vi "Read Subscribe request data JSON.vi"(8 "error in (no error)":errorcluster, 11 "Subscribe JSON in":refnum<class "Subscribe JSON.lvclass">) -> (0 "error out":errorcluster, 2 "Subscribe request data (JSON)":T1={"Topic"="", "Subscribe result notifer"=refnum, "Options"="{}"}, 3 "Subscribe JSON out":refnum<class "Subscribe JSON.lvclass">)   [LabVIEW 2020, in "wamplv.lvlib" / "Subscribe JSON.lvclass"]
uses:
  Subscribe JSON.lvclass
  Subscribe JSON.lvclass/Subscribe JSON.ctl
  WAMP Client/Private/TypeDef/EVENT payload (JSON).ctl
  wamplv.lvlib
  WAMP Client/API/TypeDefs/Error or abort detail (JSON).ctl
  WAMP Client/API/TypeDefs/Combined error.ctl
  Subscribe result (JSON).ctl
  WAMP Client/Private/TypeDef/SUBSCRIBE Request Data (JSON).ctl
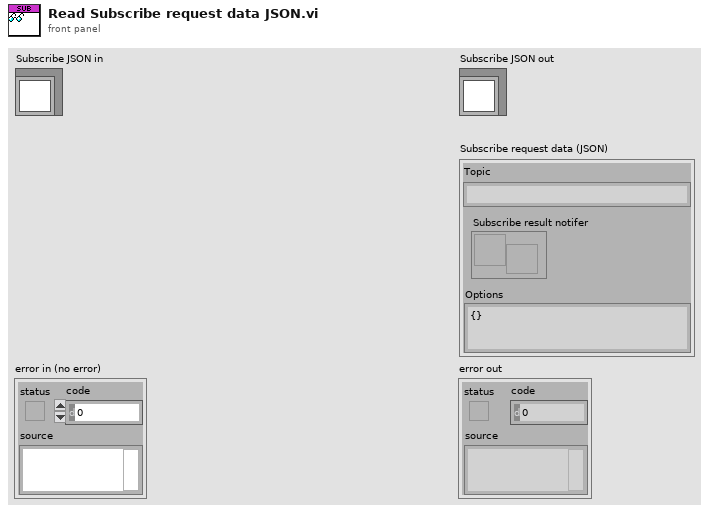
[diagram p1: front panel]
types:
  T1 = typedef "wamplv.lvlib/SUBSCRIBE Request Data (JSON).ctl" = cluster{"Topic":string, "Subscribe result notifer":refnum<notifier>, "Options":string}
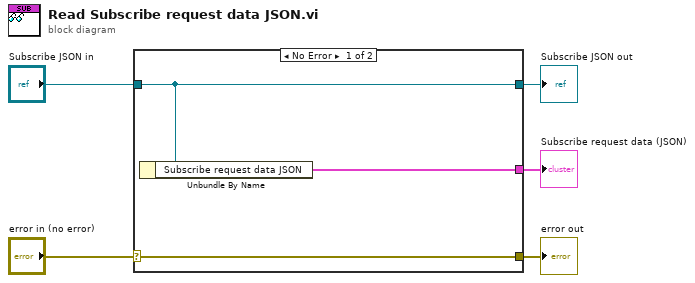
[diagram p0: block diagram]
diagram:
  n1 = case shown="No Error" "error in (no error)" {
    selector: "error in (no error)" -> [w8 w9]
    tunnel: [w8 w9] -> w4
    tunnel: [w7 w10] -> w2
    tunnel: "Subscribe JSON in" -> [w7 w10]
    tunnel: [w6 _] -> w1
    frame No Error {
      n2 = Unbundle By Name(w7) -> ("Subscribe request data JSON"=w6:T1)
    }
    frame Error {
    }
  }
  "error out" <- w4
  "Subscribe JSON out" <- w2
  "Subscribe request data (JSON)" <- w1
